vi "Find Related Particle.vi"(10 "All Reports":T1, 11 "Base Report":T1) -> (3 "Nearby":bool)   [LabVIEW 2017]
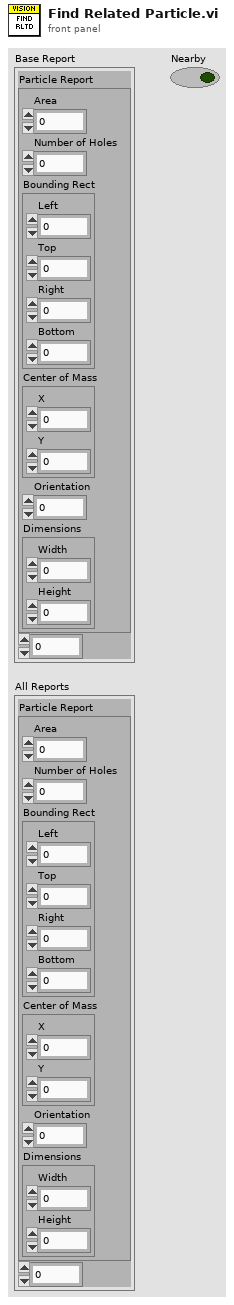
[diagram p1: front panel]
types:
  T1 = cluster{"Particle Report":cluster{"Area":dbl, "Number of Holes":dbl, "Bounding Rect":cluster{"Left":dbl, "Top":dbl, "Right":dbl, "Bottom":dbl}, "Center of Mass":cluster{"X":dbl, "Y":dbl}, "Orientation":dbl, "Dimensions":cluster{"Width":dbl, "Height":dbl}}, i32}
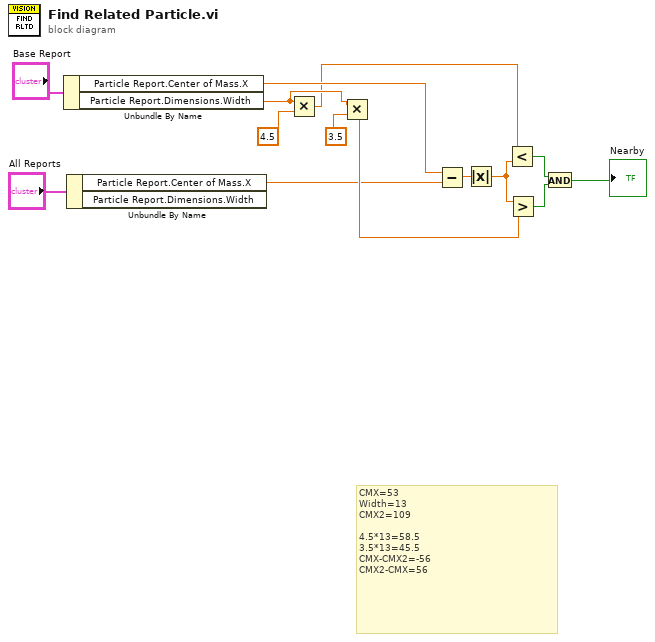
[diagram p0: block diagram]
diagram:
  # "CMX=53\nWidth=13\nCMX2=109\n\n4.5*13=58.5\n3.5*13=45.5\nCMX-CMX2=-56\nCMX2-CMX=56"
  n1 = Unbundle By Name("Base Report") -> ("Particle Report.Center of Mass.X"=w10:dbl, "Particle Report.Dimensions.Width"=w11:dbl)
  n2 = Unbundle By Name("All Reports") -> ("Particle Report.Center of Mass.X"=w1:dbl)  [unwired: 1 out]
  n3 = Multiply(x=w11, y=4.5) -> (x*y=w4:dbl)
  n4 = Multiply(x=w11, y=3.5) -> (x*y=w5:dbl)
  n5 = Subtract(x=w10, y=w1) -> ()  [unwired: 1 out]
  n6 = Absolute Value(x=w1) -> (abs(x)=w2:dbl)
  n7 = Less?(x=w4, y=w2) -> (x < y?=w7:bool)
  n8 = Greater?(x=w2, y=w5) -> (0:w6:bool)
  n9 = And(x=w7, y=w6) -> (x .and. y?=→"Nearby":bool)
